vi "10-Tap 8-bit Camera without DRAM (FPGA-SIM)no additional processing.vi"() -> ()   [LabVIEW 2013]
doc: "This is the FPGA VI for the 10-Tap 8-Bit Camera with DRAM example. This example demonstrates how to acquire images from a 10-tap, 8-bit, extended configuration, Camera Link camera and transfer the images to the host. This example supports area scan and line scan cameras for both continuous and finite acquisitions.\n\nThis example also demonstrates the use of DRAM as a frame buffer for very high speed acquisitions. Data packing and flow-control are also employed to maximize use of the available DRAM and FIFOs in terms of both memory space and performance.\n\nAdditionally, the example demonstrates the serial server, which allows third-party camera configuration utilities to communicate with the camera using the Camera Link serial interface while this VI is running."
uses:
  <vilib>/rvi/DataTransferAndStorage/Container/XNode/niFpgaContainer.xnode
  <vilib>/Platform/TimedLoop/XDataNode/XDataNode.xnode
  <vilib>/Platform/TimedLoop/XDataNode/timing_clust.ctl
  <vilib>/Platform/TimedLoop/XDataNode/XDNodeRunTimeDep.lvlib
  <vilib>/Platform/TimedLoop/XDataNode/wakeup.ctl
  <vilib>/Platform/TimedLoop/XDataNode/nitl_modes.ctl
  <vilib>/rvi/interface/RandomDataEmulation/nirviRandomDataFpgaReadWriteTemplate.vi
  FPGA/Globals/Accumulated Sector Intensity.vi
  FPGA/Globals/Pixel Location Global.vi
  FPGA/Globals/Wing Square Wave Frequency Global.vi
  FPGA/Globals/Sector Parameter Global.vi
  Common/CL Signal Mapping.ctl
  Common/CL Configuration.ctl
  FPGA/Sector/Accumulate/Sector Parameter Cluster.ctl
panel:
  out "TO Count":u32
  out "Target Sim TO":bool
  out "Cam Data Timeout":bool
  out "Host DMA Timeout":bool
  out "Number of Elements to Read Cam Data":u32
  out "Number of Elements to Write Host DMA":u32
  in  "Words per image":u32=1000
  in  "Y Resolution":u16=1000
  in  "X Resolution":u16=1000
  in  "[Average BG Intensity]":u8[](array[numeric])=[0, 0, 0, 0, 0, 0, 0, 0, 0, 0, 0, 0, 0, 0, 0, 0, 0, 0, 0, 0, 0, 0, 0, 0, 0, 0, 0, 0, 0, 0, 0, 0]
  in  "Sector Threshold":u8
  in  "# of Frames to Average":u8=1
  in  "Sector Parameters Right":T1={"Start Angle"=0.0, "End Angle"=0.4708251953125, "Inner Radius"=309, "Outter Radius"=405, "Hinge X"=685, "Hinge Y"=527, "NumWingSectors"=8}
  in  "Sector Parameters Left":T1={"Start Angle"=0.65740966796875, "End Angle"=0.99468994140625, "Inner Radius"=309, "Outter Radius"=405, "Hinge X"=464, "Hinge Y"=534, "NumWingSectors"=8}
  in  "CL Config.Configuration":T2=enum."Full"
  in  "CL Config.Signal Mapping":T3=enum."Basler 10-tap"
  in  "CL Config.Line Scan":bool
  in  "CL Config.DVAL Active High":bool=TRUE
  in  "CL Config.LVAL Active High":bool=TRUE
  in  "CL Config.FVAL Active High":bool=TRUE
  in  "CL Config.Spare Active High":bool=TRUE
  in  "Acq Control.Line Scan Height":u32
  in  "Acq Control.Frames To Acq":u32
  in  "Acq Control.Acquire":bool
  in  "Acq Control.Cancel Acq":bool
  in  "Acq Control.Ignore DVAL":bool
  in  "Acq Control.Initialize":bool
  out "Acq Status.Acq In Progress":bool
  out "Acq Status.Clocks Per Line":u32
  out "Acq Status.Frames Acq'd":u32
  out "Acq Status.Lines Per Frame":u32
  out "Acq Status.DMA Write Timeout":bool
  out "Acq Status.Initialized":bool
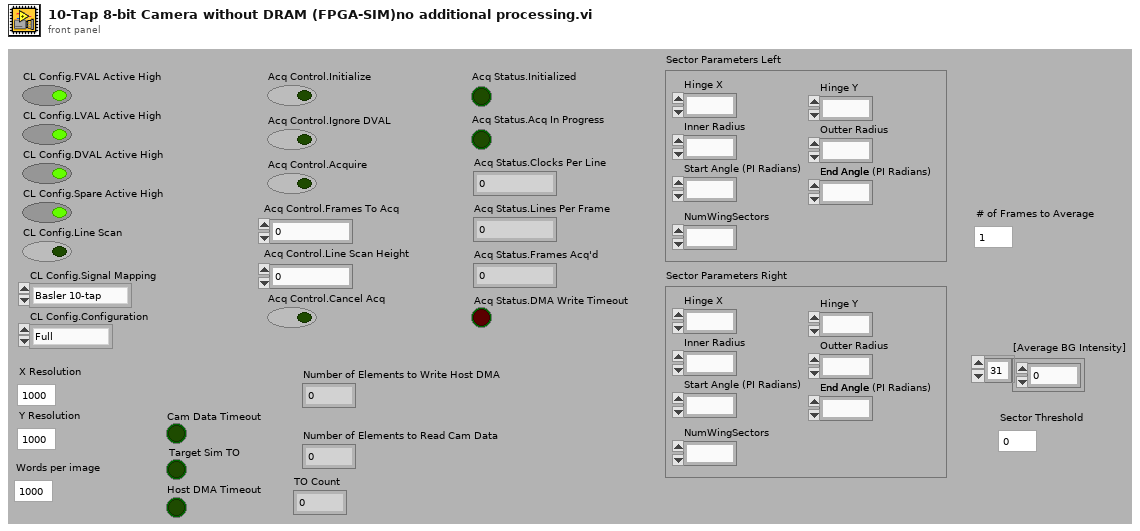
[diagram p1: front panel]
types:
  T1 = typedef "Sector Parameter Cluster.ctl" = cluster{"Start Angle":fxp<+/-,17,2>, "End Angle":fxp<+,17,3>, "Inner Radius":u16, "Outter Radius":u16, "Hinge X":u16, "Hinge Y":u16, "NumWingSectors":u8}
  T2 = typedef "CL Configuration.ctl" = enum8{"Base", "Medium", "Full"}
  T3 = typedef "CL Signal Mapping.ctl" = enum8{"Standard", "Basler 10-tap", "Vosskühler 10-tap"}
  T4 = typedef "XDNodeRunTimeDep.lvlib/timing_clust.ctl" = cluster{"Expected End [f-1]":u64, "Actual End [f-1]":u64, "Finished Late? [f-1]":bool, "Expected End [i-1]":u64, "Actual End [i-1]":u64, "Finished Late? [i-1]":bool, "Expected Start [i]":u64, "Actual Start [i]":u64, "Expected Start [f]":u64, "Actual Start [f]":u64, "Source Name":string, "Structure Name":string, "Period":i64, "Deadline":i64, "Offset":i64, "Start":i64, "Priority":i32, "Timeout":i32, "Mode":T5, "Wakeup Reason":T6, "Error":errorcluster, "Source Type":string, "Secondary Source Type":string, "Global End Time":u64, "Global Start Time":u64, "Frame Duration":u64, "Iteration Duration":u64, "Assigned CPU":i32, "I/O Scan Engine Mode":u32}
  T5 = typedef "XDNodeRunTimeDep.lvlib/nitl_modes.ctl" = enum32{"No Change", "Process missed periods, maintain original phase", "Discard missed periods, maintain original phase", "Process missed periods, ignore original phase", "Discard missed periods, ignore original phase"}
  T6 = typedef "XDNodeRunTimeDep.lvlib/wakeup.ctl" = enum32{"Normal", "Aborted", "Asynchronous wakeup", "Timing source error", "Timed loop error", "Timeout"}
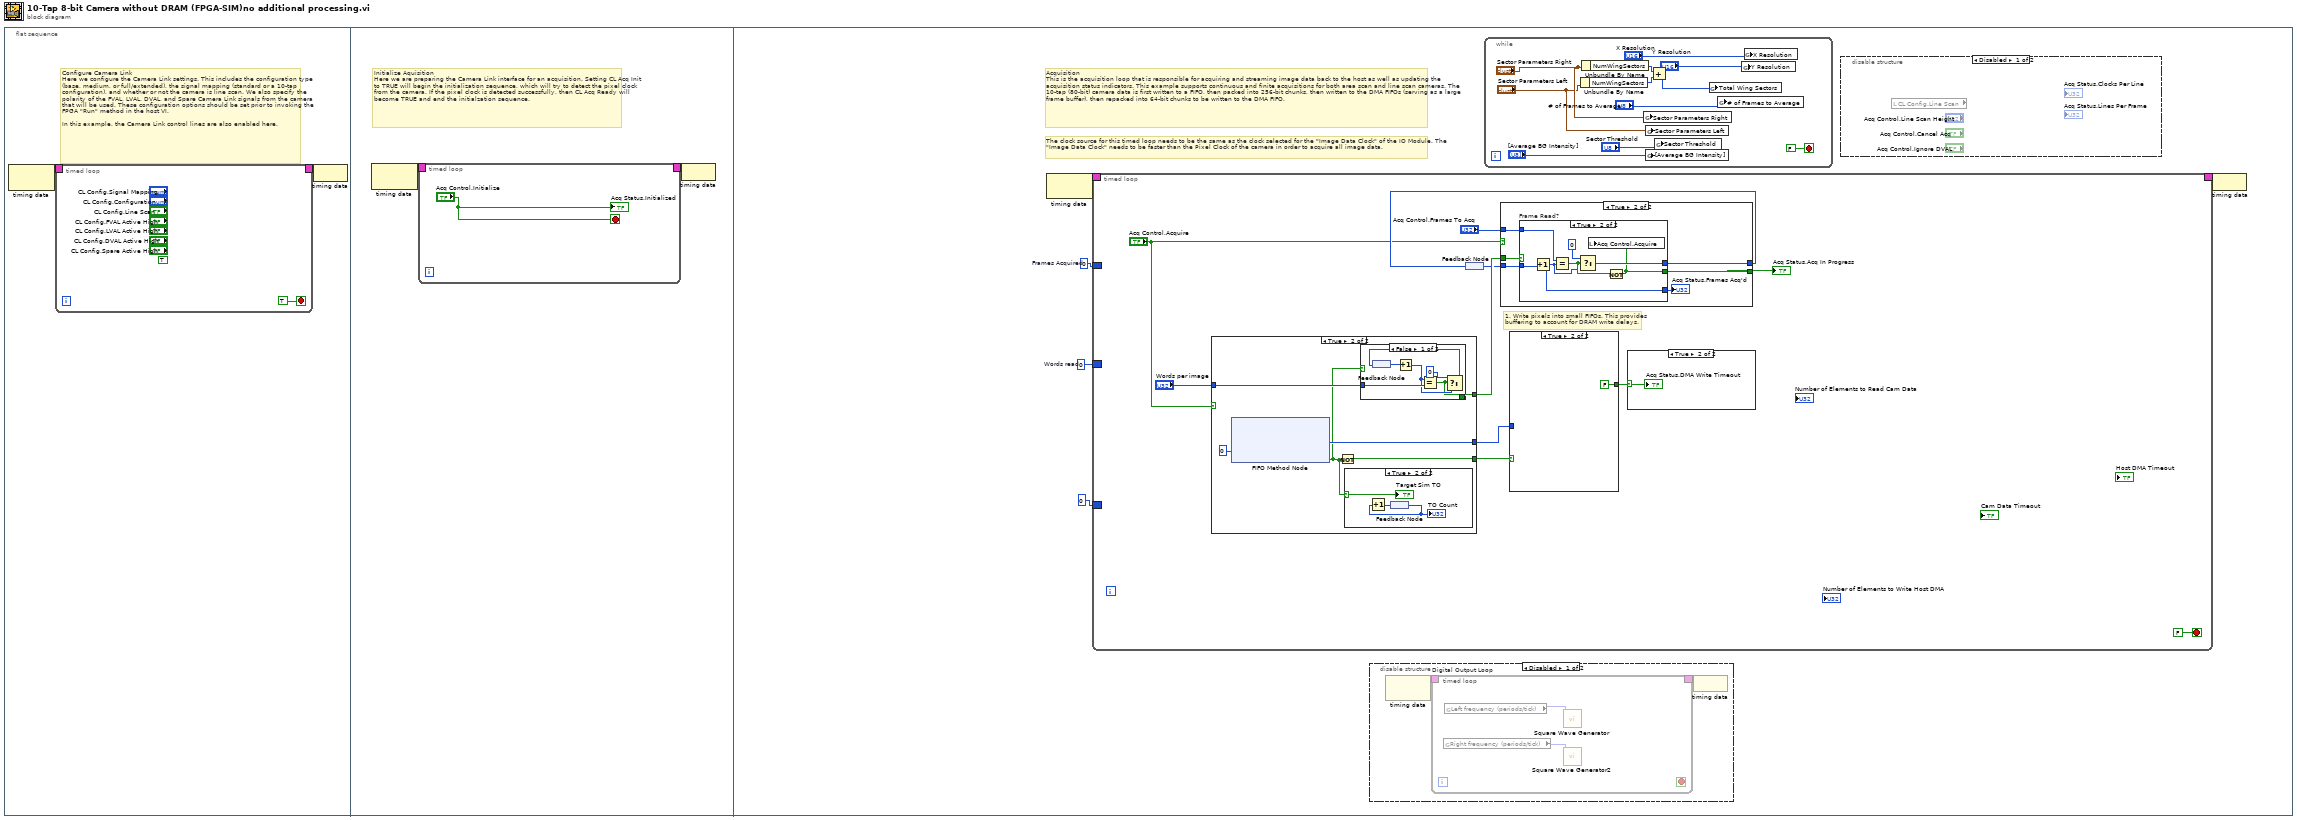
[diagram p0: block diagram]
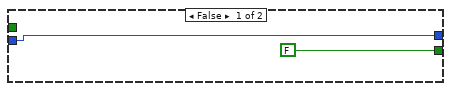
[diagram p5: hidden frame]
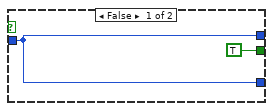
[diagram p6: hidden frame]
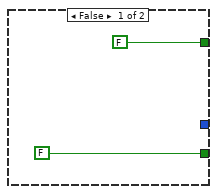
[diagram p7: hidden frame]
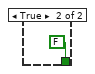
[diagram p9: hidden frame]
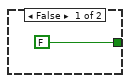
[diagram p10: hidden frame]
diagram:
  n1 = flat-sequence {
    frame #0 {
      # "Configure Camera Link\nHere we configure the Camera Link settings. This includes the configuration type (base, medium, or full/extended), the signal mapping (standard or a 10-tap configuration), and whether or not the camera is line scan. We also specify the polarity of the FVAL, LVAL, DVAL, and Spare Camera Link signals from the camera that will be used. These configuration options should be set prior to invoking the FPGA \"Run\" method in the host VI.\n\nIn this example, the Camera Link control lines are also enabled here."
      n2 = node-c288() -> (w2:T4)  [unwired: 1 in]
      n3 = timed-loop {
        timing: w2 -> [_]
        timing-out: [_] -> w1
        stop <- TRUE stop-if-true
        (unwired) TRUE ("IO Module\\CL Control Enable")
      }
      n4 = node-c288(w1) -> ()
    }
    frame #1 {
      # "Initialize Aquisition\nHere we are preparing the Camera Link interface for an acquisition. Setting CL Acq Init to TRUE will begin the initialization sequence, which will try to detect the pixel clock from the camera. If the pixel clock is detected successfully, then CL Acq Ready will become TRUE and end the initialzation sequence."
      n5 = node-c288() -> (w9:T4)  [unwired: 1 out]
      n6 = timed-loop {
        timing: w9 -> [_]
        timing-out: [_] -> w8
        stop <- "Acq Control.Initialize" stop-if-true
        "Acq Status.Initialized" <- "Acq Control.Initialize"
      }
      n7 = node-c288(w8) -> ()
    }
    frame #2 {
      w16 = u32 0  # Frames Acquired
      w17 = u32 0  # Words read
      # "The clock source for this timed loop needs to be the same as the clock selected for the \"Image Data Clock\" of the IO Module. The \"Image Data Clock\" needs to be faster than the Pixel Clock of the camera in order to acquire all image data."
      # "Acquisition\nThis is the acquisition loop that is responsible for acquiring and streaming image data back to the host as well as updating the acquisition status indicators. This example supports continuous and finite acquisitions for both area scan and line scan cameras. The 10-tap (80-bit) camera data is first written to a FIFO, then packed into 256-bit chunks, then written to the DMA FIFOs (serving as a large frame buffer), then repacked into 64-bit chunks to be written to the DMA FIFO."
      n8 = node-c288() -> (w19:T4)  [unwired: 1 in]
      n9 = timed-loop {
        timing: w19 -> [_]
        timing-out: [_] -> w18
        border: w17 -> [_]
        border: w16 -> [_]
        border: u32 0 -> [_]
        stop <- FALSE stop-if-true
        # "1. Write pixels into small FIFOs. This provides\nbuffering to account for DRAM write delays."
        n10 = case shown="True" "Acq Control.Acquire" {
          tunnel: [_ w69] -> w43
          tunnel: [FALSE w65] -> w41
          tunnel: "Words per image" -> [_ w67]
          tunnel: [FALSE w66] -> w39
          frame False {
          }
          frame True {
            n11 = xnode ("FIFO Method Node")("Timeout"=0) -> ("Element"=w69:u64, "Timed Out?"=w64:bool)  [unwired: 1 in, 1 out]
            n12 = Not(x=w64) -> (.not. x?=w65:bool)
            n13 = case shown="True" w64 {
              selector: w64 -> [_ w72]
              frame False {
              }
              frame True {
                n14 = feedback #1() -> (w70:u32)
                "TO Count" <- w70
                n15 = Increment(x=w70) -> (x+1=w71:u32)
                n16 = feedback-in #1(w71) -> ()
                "Target Sim TO" <- w72
              }
            }
            n17 = case shown="False" w64 {
              tunnel: w67 -> [w78 _]
              tunnel: [w73 FALSE] -> w66
              frame False {
                n18 = feedback #2() -> (w77:u32)
                n19 = Increment(x=w77) -> (x+1=w74:u32)
                n20 = Equal?(x=w74, y=w78) -> (x = y?=w73:bool)
                n21 = Select(t=u32 0 ("Acq Status.Frames Acq'd"), s=w73, f=w74) -> (s? t:f=w75:u32)
                n22 = feedback-in #2(w75) -> ()
              }
              frame True {
              }
            }
          }
        }
        n23 = feedback #3() -> (w38:u32)
        n24 = case shown="True" "Acq Control.Acquire" {
          tunnel: w39 -> [_ w52]
          tunnel: w38 -> [w46 w51]
          tunnel: "Acq Control.Frames To Acq" -> [_ w50]
          tunnel: [w46 w49] -> w36
          tunnel: [FALSE w48] -> w35
          frame False {
          }
          frame True {
            n25 = case "Frame Read?" shown="True" w52 {
              tunnel: w51 -> [w53 w61]
              tunnel: w50 -> [_ w60]
              tunnel: [w53 w58] -> w49
              tunnel: [TRUE w56] -> w48
              tunnel: [w53 w55] -> w47
              frame False {
              }
              frame True {
                n26 = Increment(x=w61) -> (x+1=w55:u32)
                n27 = Equal?(x=w60, y=w55) -> (x = y?=w57:bool)
                n28 = Select(t=u32 0 ("Frames Acquired"), s=w57, f=w55) -> (s? t:f=w58:u32)
                n29 = Not(x=w57) -> (.not. x?=w56:bool)
                n30 = local write "Acq Control.Acquire"(w56) -> ()
              }
            }
            "Acq Status.Frames Acq'd" <- w47
          }
        }
        "Acq Status.Acq In Progress" <- w35
        n31 = feedback-in #3(w36) -> ()
        n32 = case shown="True" w41 {
          tunnel: [FALSE ("Timed Out?") FALSE ("Timed Out?")] -> w34
          tunnel: w43 -> [_ _]
          frame False {
          }
          frame True {
          }
        }
        n33 = case shown="True" w34 {
          selector: w34 -> [_ w44]
          frame False {
          }
          frame True {
            "Acq Status.DMA Write Timeout" <- w44
          }
        }
      }
      n34 = disable-structure shown="Disabled" {
        frame Disabled {
          n35 = node-c288() -> (w26:T4)  [unwired: 1 in]
          n36 = timed-loop "Digital Output Loop" {
            timing: w26 -> [_]
            timing-out: [_] -> w25
            stop <- _ stop-if-true
            n37 = global read "Wing Square Wave Frequency Global.vi" "Right frequency (periods/tick)"() -> (w27:fxp<+,32,0>)
            n38 = global read "Wing Square Wave Frequency Global.vi" "Left frequency (periods/tick)"() -> (w28:fxp<+,32,0>)
            n39 = call "Square Wave Generator"("frequency (periods/tick)"=w28) -> ()  [unwired: 14 in, 1 out]
            n40 = call "Square Wave Generator2"("frequency (periods/tick)"=w27) -> ()  [unwired: 14 in, 1 out]
          }
          n41 = node-c288(w25) -> ()
        }
        frame Enabled {
        }
      }
      n42 = while {
        stop <- FALSE stop-if-true
        n43 = Unbundle By Name("Sector Parameters Left") -> ("NumWingSectors"=w94:u8)
        n44 = Unbundle By Name("Sector Parameters Right") -> ("NumWingSectors"=w95:u8)
        n45 = global write "Sector Parameter Global.vi" "Sector Parameters Right"("Sector Parameters Right") -> ()
        n46 = global write "Sector Parameter Global.vi" "Sector Parameters Left"("Sector Parameters Left") -> ()
        n47 = global write "Sector Parameter Global.vi" "[Average BG Intensity]"("[Average BG Intensity]") -> ()
        n48 = Add(x=w95, y=w94) -> (x+y=w93:u8)
        n49 = global write "Sector Parameter Global.vi" "Sector Threshold"("Sector Threshold") -> ()
        n50 = global write "Accumulated Sector Intensity.vi" "Total Wing Sectors"(w93) -> ()
        n51 = global write "Pixel Location Global.vi" "# of Frames to Average"("# of Frames to Average") -> ()
        n52 = global write "Pixel Location Global.vi" "Y Resolution"("Y Resolution") -> ()
        n53 = global write "Pixel Location Global.vi" "X Resolution"("X Resolution") -> ()
      }
      n54 = disable-structure shown="Disabled" {
        frame Disabled {
          n55 = local read "CL Config.Line Scan"() -> (w22:bool)
        }
        frame Enabled {
        }
      }
      n56 = node-c288(w18) -> ()
    }
  }
